vi "Error_Logger.vi"(11 "Error_In":errorcluster) -> (4 "Error_Table":string[][](table) caption="Error Table", 15 "Error_Out":errorcluster)   [LabVIEW 2021]
doc: "This VI Shows the Error data of current and temperature."
uses:
  Controls/Queue_Operation_Select.ctl
  Controls/Error_Data.ctl
  Controls/State_and_Data.ctl
  Controls/Timer_Select.ctl
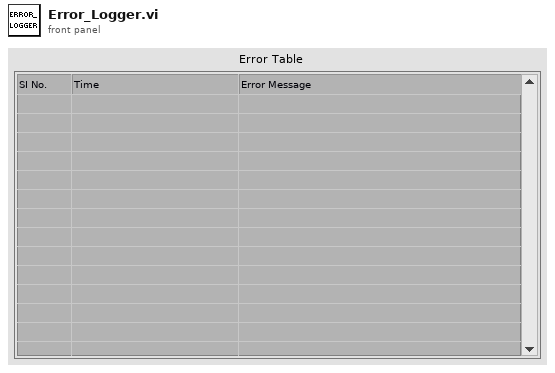
[diagram p1: front panel]
types:
  T1 = typedef "Timer_Select.ctl" = enum16{"Start_Timer", "Time_Out?", "Stop_Timer"}
  T2 = typedef "State_and_Data.ctl" = cluster{"State":string, "Data":variant}
  T3 = typedef "Queue_Operation_Select.ctl" = enum16{"Obtain_Queue", "Enqueue", "Enqueue_First", "Enqueue_N", "Lossy_Enqueue", "Preview", "Queue_Status", "Dequeue", "Flush", "Release_Queue"}
  T4 = enum32{"Invalid", "Standard", "Closed", "Hidden", "Minimized", "Maximized"}
  T5 = typedef "Error_Data.ctl" = cluster{"Error_Table_Data":string[][], "SI_No":i32, "Log_Rate":u32}
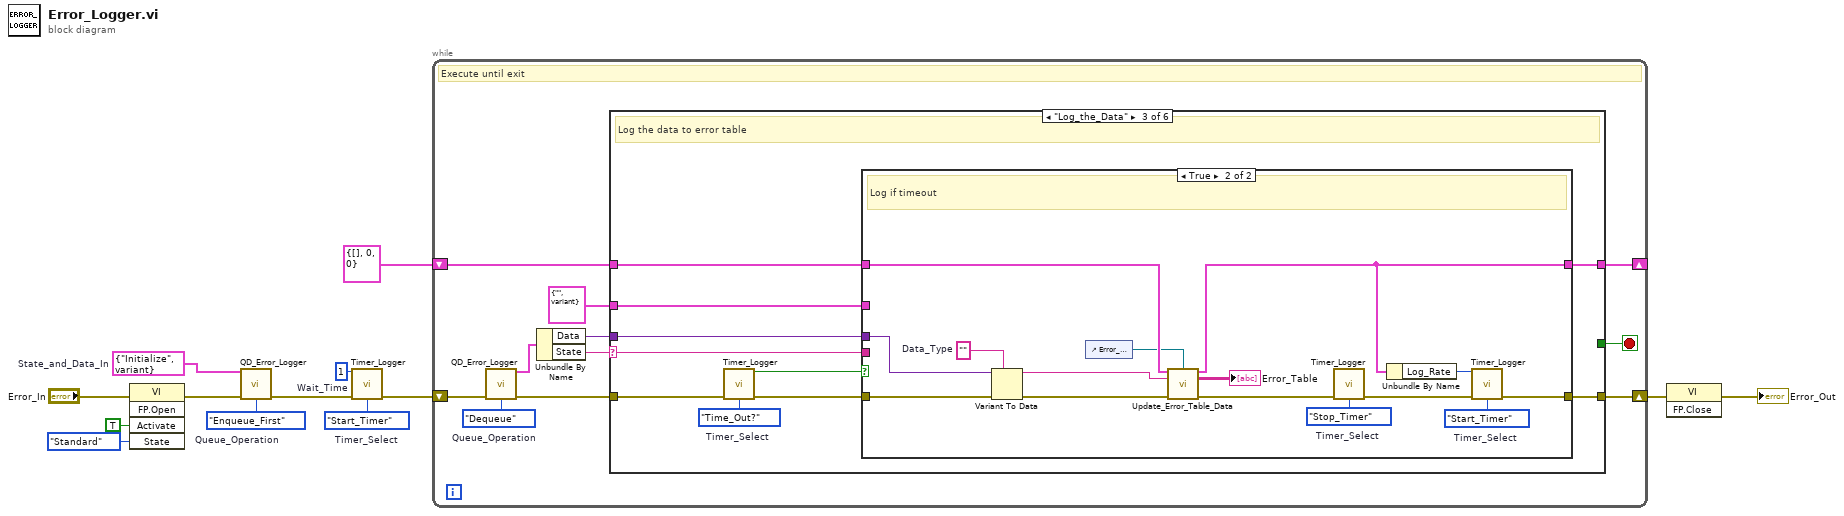
[diagram p0: block diagram]
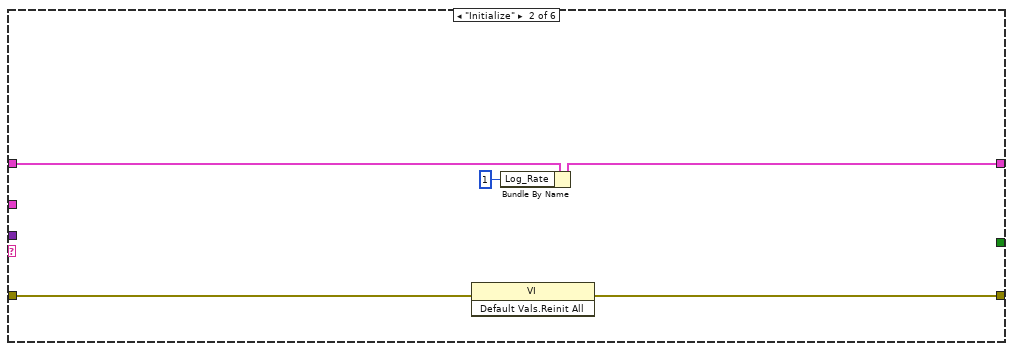
[diagram p3: hidden frame]
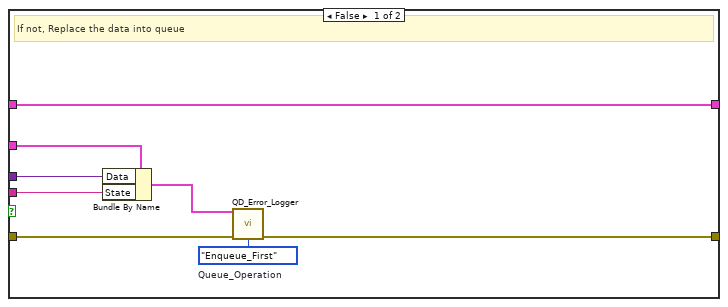
[diagram p4: hidden frame]
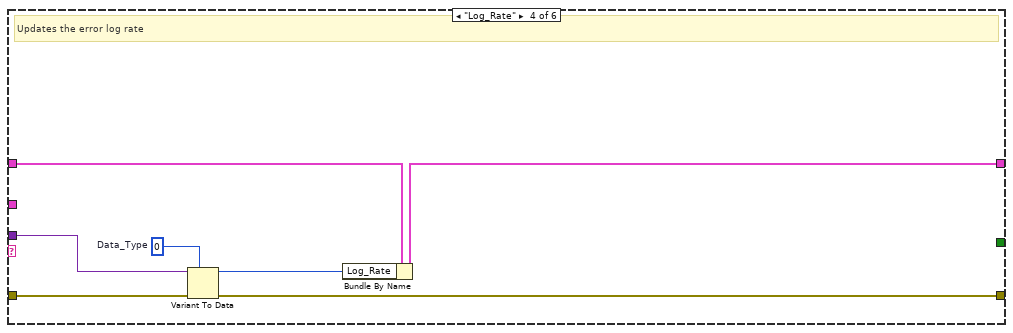
[diagram p5: hidden frame]
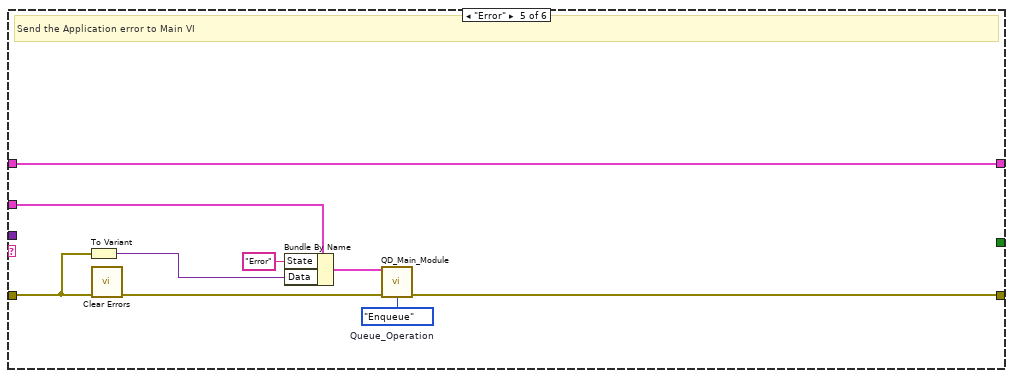
[diagram p6: hidden frame]
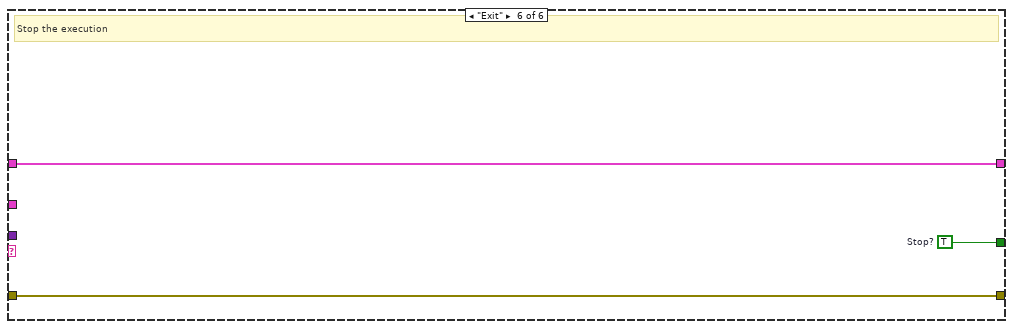
[diagram p7: hidden frame]
diagram:
  w1 = u32 1  # Wait_Time
  w2 = Timer_Select."Start_Timer"  # Timer_Select
  w4 = T2 {"State"="Initialize", "Data"=variant}  # State_and_Data_In
  w5 = Queue_Operation_Select."Enqueue_First"  # Queue_Operation
  n1 = invoke class="VI" method="FP.Open"(error in="Error_In", "Activate"=TRUE ("Activate?"), "State"=T4."Standard") -> (error out=w7:errorcluster)  [unwired: 2 in, 4 out]
  n2 = call "QD_Error_Logger.vi"("State_and_Data_In"=w4, "Error_In"=w7, "Queue_Operation"=w5) -> ("Error_Out"=w6:errorcluster)  [unwired: 11 in, 1 out]
  n3 = call "Timer_Logger.vi"("Wait_Time"=w1, "Error_In"=w6, "Timer_Select"=w2) -> ("Error_Out"=w3:errorcluster)  [unwired: 11 in, 1 out]
  n4 = while {
    shift-right: [w23] -> _
    shift-left: T5 {"Error_Table_Data"=[], "SI_No"=0, "Log_Rate"=0} -> [w24]
    shift-right: [w14] -> w11
    shift-left: w3 -> [w15]
    stop <- w22 stop-if-true
    w18 = Queue_Operation_Select."Dequeue"  # Queue_Operation
    # "Execute until exit"
    n5 = call "QD_Error_Logger.vi"("Error_In"=w15, "Queue_Operation"=w18) -> ("State_and_Data_Out"=w17:T2, "Error_Out"=w19:errorcluster)  [unwired: 12 in]
    n6 = Unbundle By Name(w17) -> ("Data"=w20:variant, "State"=w21:string)
    n7 = case shown="\"Log_the_Data\"" w21 {
      selector: w21 -> [_ _ w35 _ _ _]
      tunnel: w24 -> [w26 w31 w37 w70 w80 w83]
      tunnel: [w26 w30 w41 w69 w80 w83] -> w23
      tunnel: [w25 w27 w40 w68 w73 w82] -> w14
      tunnel: w19 -> [w25 w28 w39 w71 w74 w82]
      tunnel: w20 -> [_ _ w38 w67 _ _]
      tunnel: T2 {"State"="", "Data"=variant} ("State_and_Data_In") -> [_ _ w36 _ w72 _]
      tunnel: [_ _ _ _ _ w81] -> w22
      frame Default {
      }
      frame "Initialize" {
        n8 = invoke class="VI" method="Default Vals.Reinit All"(error in=w28) -> (error out=w27:errorcluster)  [unwired: 2 in, 2 out]
        n9 = Bundle By Name(cluster=w31, "Log_Rate"=u32 1) -> (w30:T5)
      }
      frame "Log_the_Data" {
        w32 = Timer_Select."Time_Out?"  # Timer_Select
        # "Log the data to error table"
        n10 = call "Timer_Logger.vi"("Error_In"=w39, "Timer_Select"=w32) -> ("Time_Out?"=w33:bool, "Error_Out"=w34:errorcluster)  [unwired: 12 in]
        n11 = case shown="True" w33 {
          tunnel: [w48 w51] -> w41
          tunnel: [w47 w53] -> w40
          tunnel: w34 -> [w49 w63]
          tunnel: w38 -> [w44 w62]
          tunnel: w37 -> [w48 w59]
          tunnel: w36 -> [w45 _]
          tunnel: w35 -> [w43 _]
          frame False {
            w46 = Queue_Operation_Select."Enqueue_First"  # Queue_Operation
            # "If not, Replace the data into queue"
            n12 = Bundle By Name(cluster=w45, "Data"=w44, "State"=w43) -> (w42:T2)
            n13 = call "QD_Error_Logger.vi"("State_and_Data_In"=w42, "Error_In"=w49, "Queue_Operation"=w46) -> ("Error_Out"=w47:errorcluster)  [unwired: 11 in, 1 out]
          }
          frame True {
            w52 = Timer_Select."Start_Timer"  # Timer_Select
            w54 = Timer_Select."Stop_Timer"  # Timer_Select
            w61 = ""  # Data_Type
            # "Log if timeout"
            n14 = Variant To Data(error in=w63, type=w61, Variant=w62) -> (data=w60:string, error out=w56:errorcluster)
            n15 = control-ref of="Error_Table"() -> (w57:refnum<vi>)
            n16 = call "Update_Error_Table_Data.vi"("Error_Data_In"=w59, "Table_Reference"=w57, "Error_Message"=w60, "Error_In"=w56) -> ("Error_Data_Out"=w51:T5, "Error_Table_Data"=→"Error_Table":string[][], "Error_Out"=w64:errorcluster)  [unwired: 9 in]
            n17 = call "Timer_Logger.vi"("Error_In"=w64, "Timer_Select"=w54) -> ("Error_Out"=w55:errorcluster)  [unwired: 12 in, 1 out]
            n18 = Unbundle By Name(w51) -> ("Log_Rate"=w50:u32)
            n19 = call "Timer_Logger.vi"("Wait_Time"=w50, "Error_In"=w55, "Timer_Select"=w52) -> ("Error_Out"=w53:errorcluster)  [unwired: 11 in, 1 out]
          }
        }
      }
      frame "Log_Rate" {
        w66 = u32 0  # Data_Type
        # "Updates the error log rate"
        n20 = Variant To Data(error in=w71, type=w66, Variant=w67) -> (data=w65:u32, error out=w68:errorcluster)
        n21 = Bundle By Name(cluster=w70, "Log_Rate"=w65) -> (w69:T5)
      }
      frame "Error" {
        w79 = Queue_Operation_Select."Enqueue"  # Queue_Operation
        # "Send the Application error to Main VI"
        n22 = To Variant(anything=w74) -> (Variant=w76:variant)
        n23 = call <vilib>:"Clear Errors.vi"("error in (no error)"=w74) -> ("error out"=w75:errorcluster)  [unwired: 5 in, 1 out]
        n24 = Bundle By Name(cluster=w72, "State"="Error", "Data"=w76) -> (w78:T2)
        n25 = call "QD_Main_Module.vi"("Data_In"=w78, "Error_In"=w75, "Queue_Operation"=w79) -> ("Error_Out"=w73:errorcluster)  [unwired: 10 in, 2 out]
      }
      frame "Exit" {
        w81 = TRUE  # Stop?
        # "Stop the execution"
      }
    }
  }
  n26 = invoke class="VI" method="FP.Close"(error in=w11) -> (error out=→"Error_Out":errorcluster)  [unwired: 2 in, 2 out]
